vi "MessageServiceCallbackInternal.vi"(4 "MessageWithState":refnum<user-event>, 5 "Event Data":cluster{"sender":refnum<k24>, "e":refnum<k24>}, 6 "Control Ref":refnum<k24>, 7 "Event Common Data":T1) -> ()   [LabVIEW 2017]
uses:
  C:/Program Files (x86)/National Instruments/LabVIEW 2017/vi.lib/addons/InsightCM/Binaries/LabviewMessageAdapter.dll
  Binaries/LabviewMessageAdapter.dll
  <vilib>/addons/InsightCM/MessageBus/Base/controls/MessageWithState.ctl
  <vilib>/addons/InsightCM/MessageBus/Base/controls/Message.ctl
  <vilib>/addons/InsightCM/MessageBus/Base/controls/MessageHeader.ctl
  <vilib>/addons/InsightCM/MessageBus/Base/controls/KeyValuePair.ctl
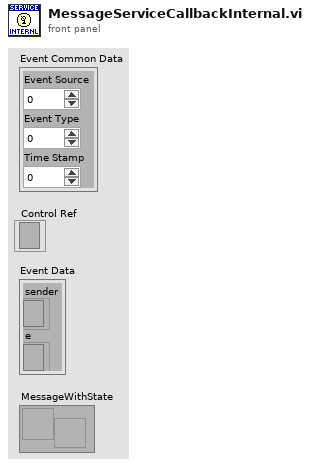
[diagram p1: front panel]
types:
  T1 = cluster{"Event Source":i32, "Event Type":u32, "Time Stamp":u32}
  T2 = typedef "MessageWithState.ctl" = cluster{"Message":T3, "State":string}
  T3 = typedef "Message.ctl" = cluster{"Header":T4, "Body":u8[]}
  T4 = typedef "MessageHeader.ctl" = cluster{"MessageName":string, "Timestamp":i64, "CorrelationId":string, "ContentType":string, "RoutingKey":string, "Properties":T5[]}
  T5 = typedef "KeyValuePair.ctl" = cluster{"Key":string, "Value":string}
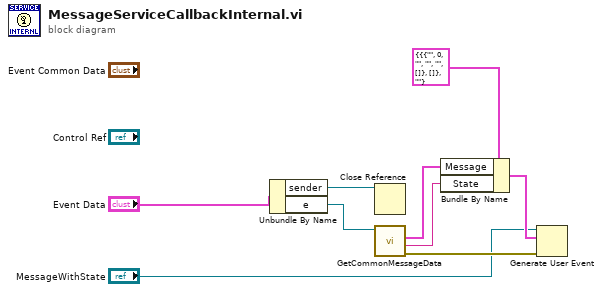
[diagram p0: block diagram]
diagram:
  n1 = Unbundle By Name("Event Data") -> ("sender"=w3:refnum<k24>, "e"=w4:refnum<k24>)
  n2 = Close Reference(reference=w3) -> ()  [unwired: 1 in, 1 out]
  n3 = call <vilib>:"GetCommonMessageData.vi"("MessageArgs"=w4) -> ("error out"=w5:errorcluster, "State"=w8:string, "Message"=w7:T3)  [unwired: 8 in]
  n4 = Bundle By Name(cluster=T2 {"Message"={"Header"={"MessageName"="", "Timestamp"=0, "CorrelationId"="", "ContentType"="", "RoutingKey"="", "Properties"=[]}, "Body"=[]}, "State"=""} ("MessageWithState"), "Message"=w7, "State"=w8) -> (w9:T2)
  n5 = Generate User Event(user event="MessageWithState", event data cluster=w9, error in=w5) -> ()  [unwired: 1 in, 2 out]
